vi "Config Init.vi"(2 "error in (no error)":errorcluster) -> (0 "error out":errorcluster, 1 "Instrument":string[](array[string]))   [LabVIEW 2018]
uses:
  Type Defs/Open IPF.ctl
  Type Defs/RT Command.ctl
  Type Defs/Global Action.ctl
  <vilib>/Utility/config.llb/Read Key (I32).vi
  <vilib>/Utility/config.llb/Read Key (Boolean).vi
  FGVs/Global Variables.vi
  <vilib>/Utility/config.llb/Read Key (String).vi
  <vilib>/Utility/config.llb/Write Key (String).vi
  <vilib>/Utility/config.llb/NI_LVConfig.lvlib
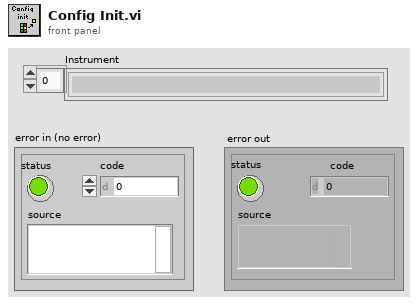
[diagram p1: front panel]
types:
  T1 = typedef "Global Action.ctl" = enum16{"Write", "Read"}
  T2 = typedef "RT Command.ctl" = enum16{"xml Start Run", "xml Start Actual Run", "xml Stop Run", "xml Runtime Update", "xml Get Status", "xml Get Table", "xml Set Table", "xml Get Configuration", "xml System Status", "xml Set LC Input Logic", "xml Get Data", "xml Get Info", "Start", "StartActualRun", "Stop", "Runtime Update", "Get Data", "Get Info", "Get Status", "Get Param", "Get Config", "Get Table", "Read ADC", "Set Oscillator", "Update Config", "Update Table", "Set All Pol", "Set Pol and DC", "Set Max Mass", "Toggle RP", "Toggle EL", "Set PIC", "Initialize Turbo", "Send Turbo Comm", "Close Turbo", "P1", "P2", "P3", "Send Serial", "Set LC Out", "Get LC In", "Read VAC", "Test Table", "Toggle Power", "Get Startup", "Set Startup", "Get ADC Table", "Set ADC Table", "Get Brief Status", "Get Detail Status", "Auxiliary Update", "Set CC Logics", "Set CC Input Logics", "Ignore Error", "invalid"}
  T3 = typedef "Open IPF.ctl" = enum16{"Init", "Create IPF"}
  T4 = typedef "NI_LVConfig.lvlib/Config Data RefNum.ctl" = refnum<k1>
  T5 = typedef "Global Configrations.ctl" = cluster{"Model Name":enum16{"QSight 110", "QSight 120", "QSight 210", "QSight 220", "QSight 410", "QSight 420", "IONICS 3Q 110", "IONICS 3Q 120", "IONICS 3Q 210", "IONICS 3Q 220", "IONICS 3Q 310", "IONICS 3Q 320", "Simulation (Single Source)", "Simulation (Dual Source)"}, "RunType":u16, "Acquisition State":enum16{"Ready", "Busy", "Waiting"}, "InstrState":enum16{"Initializing", "Mass Spectrometer is Off", "Starting Up", "Turning Power Off", "Going to Standby", "Roughing Pump Ready", "Turning Turbo Off", "Turbo Startup", "Turbopump Ready", "Checking Vacuum", "Going to Ready", "Ready", "Running", "Source Standby", "Lost Communication", "Shutting Down", "Fault", "24V Standby", "Go to 24V Standby", "Turbopump Ready-Waiting"}, "Run Mode":enum16{"MRM (Q1/Q2)", "Q1 Scan", "Q1 SRM", "Q2 Scan", "Q2 SRM", "Product Scan", "Precursor Scan", "Neutral Loss", "Neutral Gain"}, "Configration":T6, "TCP ID":refnum<k5>, "DT":bool, "Dead Time (nS)":i32, "Single Source":bool, "ADC Tables":T8[], "FW Udate":bool, "Simulator":bool}
  T6 = typedef "Configration.ctl" = cluster{"Table":T7[], "Instrument":string[]}
  T7 = typedef "_RT Configuration 2.ctl" = cluster{"Name":string, "Ch#":u8, "Min":dbl, "Max":dbl, "Def+":dbl, "Def-":dbl, "Offset":dbl, "Slope":dbl, "Type":u8, "Description":string, "SettleT":dbl}
  T8 = typedef "ADC Table.ctl" = cluster{"Name":string, "Ch#":u8, "Min":dbl, "Max":dbl, "Def+":dbl, "Def-":dbl, "Offset":dbl, "Slope":dbl, "Type":u8, "Description":string, "SettleT":dbl}
  T9 = typedef "Instrument Model.ctl" = enum16{"QSight 110", "QSight 120", "QSight 210", "QSight 220", "QSight 410", "QSight 420", "IONICS 3Q 110", "IONICS 3Q 120", "IONICS 3Q 210", "IONICS 3Q 220", "IONICS 3Q 310", "IONICS 3Q 320", "Simulation (Single Source)", "Simulation (Dual Source)"}
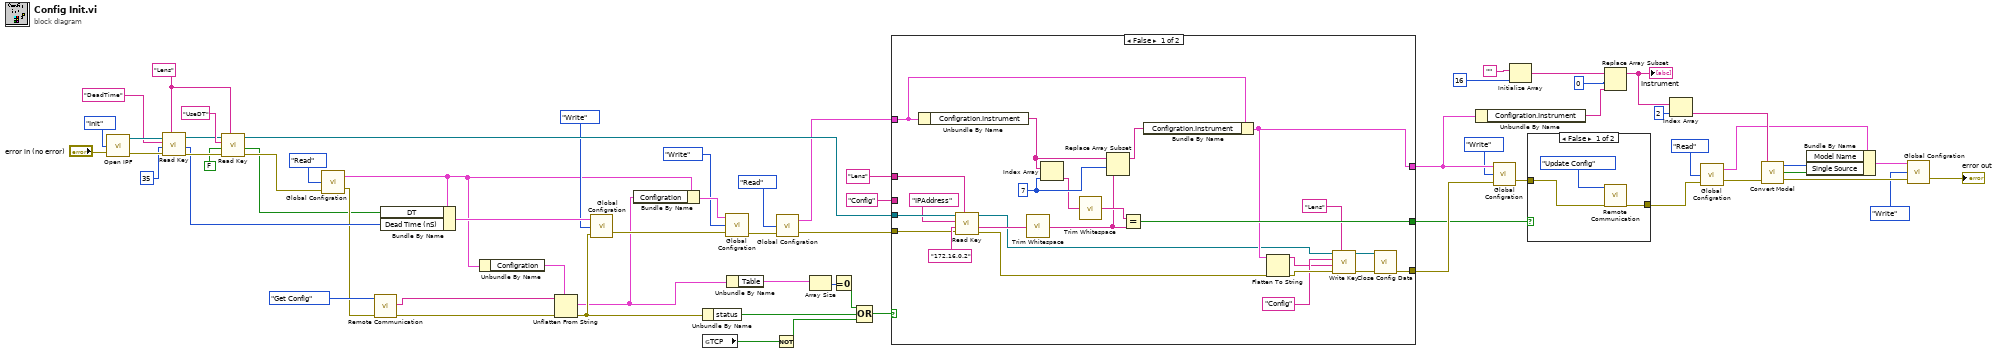
[diagram p0: block diagram]
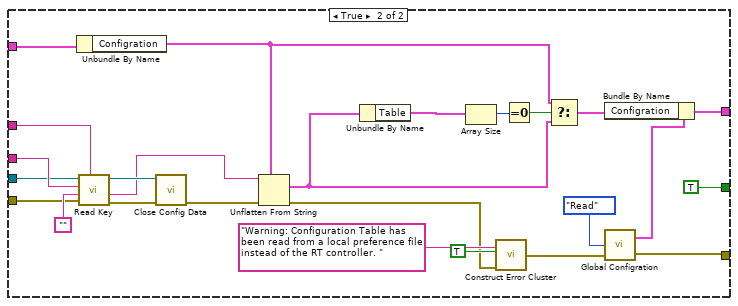
[diagram p3: hidden frame]
diagram:
  w62 = "Lens" ("section")
  n1 = call "Open IPF.vi"("Error In"="error in (no error)", 4:Open_IPF."Init") -> ("Error Out"=w64:errorcluster, "IPF refnum"=w63:T4)  [unwired: 1 in, 1 out]
  n2 = call-poly <vilib>:"Read Key.vi"("section"=w62, "error in (no error)"=w64, "default value"=35, "key"="DeadTime", "refnum"=w63) -> ("error out"=w57:errorcluster, "value"=w55:i32, "refnum out"=w58:T4)  [unwired: 4 out]
  n3 = call-poly <vilib>:"Read Key.vi"("section"=w62, "error in (no error)"=w57, "default value"=FALSE, "key"="UseDT", "refnum"=w58) -> ("error out"=w14:errorcluster, "value"=w5:bool, "refnum out"=w41:T4)  [unwired: 4 out]
  n4 = call "Global Configration.vi"("Error In"=w14, "Action"=Global_Action."Read") -> ("Error Out"=w13:errorcluster, "Parameters Out"=w9:T5)  [unwired: 1 in]
  n5 = call "Remote Communication.vi"("Error In"=w13, "Command"=RT_Command."Get Config") -> ("Error Out"=w51:errorcluster, "Info"=w52:string)  [unwired: 4 in, 2 out]
  n6 = Bundle By Name(cluster=w9, "DT"=w5, "Dead Time (nS)"=w55) -> (w54:T5)
  n7 = Unbundle By Name(w9) -> ("Configration"=w21:T6)
  n8 = Unflatten From String(type=w21, binary string=w52, error in (no error)=w51) -> (value=w8:T6, error out=w50:errorcluster)  [unwired: 3 out]
  n9 = call "Global Configration.vi"("Error In"=w50, "Action"=Global_Action."Write", "Parameters In"=w54) -> ("Error Out"=w11:errorcluster)  [unwired: 1 out]
  n10 = Bundle By Name(cluster=w9, "Configration"=w8) -> (w7:T5)
  n11 = Unbundle By Name(w50) -> ("status"=w46:bool)
  n12 = global read "Global Variables.vi" "TCP"() -> (w45:bool)
  n13 = call "Global Configration.vi"("Error In"=w11, "Action"=Global_Action."Write", "Parameters In"=w7) -> ("Error Out"=w2:errorcluster)  [unwired: 1 out]
  n14 = Unbundle By Name(w8) -> ("Table"=w48:T7[])
  n15 = Not(x=w45) -> (.not. x?=w12:bool)
  n16 = call "Global Configration.vi"("Error In"=w2, "Action"=Global_Action."Read") -> ("Error Out"=w4:errorcluster, "Parameters Out"=w3:T5)  [unwired: 1 in]
  n17 = Array Size(array=w48) -> (size(s)=w49:i32)
  n18 = Equal To 0?(x=w49) -> (x = 0?=w47:bool)
  n19 = Compound Arithmetic op=OR(w47, w46, w12) -> (w44:bool)
  n20 = case shown="False" w44 {
    tunnel: "Lens" ("section") -> [w88 w113]
    tunnel: "Config" ("section") -> [_ w112]
    tunnel: w41 -> [w89 w111]
    tunnel: [w73 w92] -> w39
    tunnel: [w78 w94] -> w40
    tunnel: [w76 TRUE] -> w25
    tunnel: w4 -> [w75 w90]
    tunnel: w3 -> [w74 w91]
    frame False {
      w84 = 7 ("index")
      n21 = Unbundle By Name(w74) -> ("Configration.Instrument"=w82:string[])
      n22 = call-poly <vilib>:"Read Key.vi"("section"=w88, "error in (no error)"=w75, "default value"="172.16.0.2", "key"="IPAddress" ("section"), "refnum"=w89) -> ("error out"=w77:errorcluster, "value"=w85:string, "refnum out"=w67:T4)  [unwired: 1 in, 3 out]
      n23 = call <vilib>:"Trim Whitespace.vi"("string"=w85) -> ("trimmed string"=w79:string)  [unwired: 1 in]
      n24 = Index Array(array=w82, index=w84) -> (element=w81:string)
      n25 = call <vilib>:"Trim Whitespace.vi"("string"=w81) -> ("trimmed string"=w83:string)  [unwired: 1 in]
      n26 = Replace Array Subset(array=w82, new element=w79, index=w84) -> (w80:string[])
      n27 = Equal?(x=w83, y=w79) -> (x = y?=w76:bool)
      n28 = Bundle By Name(cluster=w74, "Configration.Instrument"=w80) -> (w73:T5)
      n29 = Flatten To String(anything=w73, error in (no error)=w77) -> (data string=w68:string, error out=w70:errorcluster)  [unwired: 3 out]
      n30 = call-poly <vilib>:"Write Key.vi"("section"="Lens", "error in (no error)"=w70, "value"=w68, "key"="Config" ("section"), "refnum"=w67) -> ("error out"=w71:errorcluster, "refnum out"=w66:T4)  [unwired: 1 in, 4 out]
      n31 = call <vilib>:"Close Config Data.vi"("error in (no error)"=w71, "refnum"=w66) -> ("error out"=w78:errorcluster)  [unwired: 8 in, 1 out]
    }
    frame True {
      n32 = Unbundle By Name(w91) -> ("Configration"=w98:T6)
      n33 = call-poly <vilib>:"Read Key.vi"("section"=w113, "error in (no error)"=w90, "default value"="", "key"=w112, "refnum"=w111) -> ("error out"=w102:errorcluster, "value"=w100:string, "refnum out"=w103:T4)  [unwired: 1 in, 3 out]
      n34 = call <vilib>:"Close Config Data.vi"("error in (no error)"=w102, "refnum"=w103) -> ("error out"=w101:errorcluster)  [unwired: 8 in, 1 out]
      n35 = Unflatten From String(type=w98, binary string=w100, error in (no error)=w101) -> (value=w105:T6, error out=w104:errorcluster)  [unwired: 3 out]
      n36 = Unbundle By Name(w105) -> ("Table"=w106:T7[])
      n37 = Array Size(array=w106) -> (size(s)=w108:i32)
      n38 = call "Construct Error Cluster.vi"("Error In"=w104, "Reason"="Warning: Configuration Table has been read from a local preference file instead of the RT controller. ", "Call Chain"=TRUE) -> ("Error Out"=w95:errorcluster)  [unwired: 1 in]
      n39 = Equal To 0?(x=w108) -> (x = 0?=w107:bool)
      n40 = Select(t=w98, s=w107, f=w105) -> (s? t:f=w97:T6)
      n41 = call "Global Configration.vi"("Error In"=w95, "Action"=Global_Action."Read") -> ("Error Out"=w94:errorcluster, "Parameters Out"=w93:T5)  [unwired: 1 in]
      n42 = Bundle By Name(cluster=w93, "Configration"=w97) -> (w92:T5)
    }
  }
  n43 = Unbundle By Name(w39) -> ("Configration.Instrument"=w33:string[])
  n44 = call "Global Configration.vi"("Error In"=w40, "Action"=Global_Action."Write", "Parameters In"=w39) -> ("Error Out"=w24:errorcluster)  [unwired: 1 out]
  n45 = Initialize Array("", 16 ("dimension size")) -> (w35:string[])
  n46 = case shown="False" w25 {
    tunnel: w24 -> [w116 w118]
    tunnel: [w115 w118] -> w20
    frame False {
      n47 = call "Remote Communication.vi"("Error In"=w116, "Command"=RT_Command."Update Config") -> ("Error Out"=w115:errorcluster)  [unwired: 4 in, 3 out]
    }
    frame True {
    }
  }
  n48 = Replace Array Subset(array=w35, new element=w33, index=0) -> (w31:string[])
  "Instrument" <- w31
  n49 = Index Array(array=w31, index=2) -> (element=w30:string)
  n50 = call "Global Configration.vi"("Error In"=w20, "Action"=Global_Action."Read") -> ("Error Out"=w19:errorcluster, "Parameters Out"=w18:T5)  [unwired: 1 in]
  n51 = call "Convert Model.vi"("error in (no error)"=w19, "Model"=w30) -> ("error out"=w27:errorcluster, "SingleSource"=w29:bool, "Model Name  Out"=w28:T9)  [unwired: 1 in]
  n52 = Bundle By Name(cluster=w18, "Model Name"=w28, "Single Source"=w29) -> (w17:T5)
  n53 = call "Global Configration.vi"("Error In"=w27, "Action"=Global_Action."Write", "Parameters In"=w17) -> ("Error Out"=→"error out":errorcluster)  [unwired: 1 out]
